vi "Remove Danger Move Options.vi"(5 "Danger Directions":T1[](array[typedef]), 7 "Danger View":i32[](array[numeric]), 10 "Danger Threshold":i32, 11 "Direction List":T1[](array[typedef])) -> (2 "Danger":bool, 3 "Safe Directions Out":T1[](array[typedef]))   [LabVIEW 2017, in "AntFarm_MB.lvclass"]
uses:
  AntFarm_MB.lvclass
  Type Defs/Direction Enum.ctl
  Type Defs/SB Type Defs.lvlib
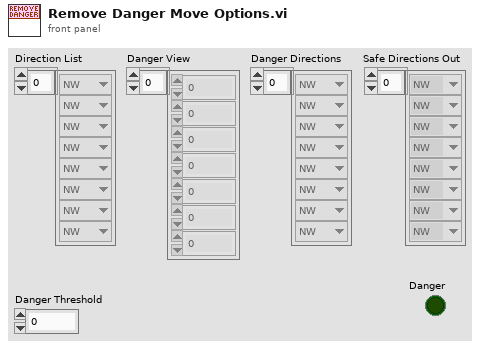
[diagram p1: front panel]
types:
  T1 = typedef "SB Type Defs.lvlib/Direction Enum.ctl" = enum16{"NW", "N", "NE", "E", "SE", "S", "SW", "W"}
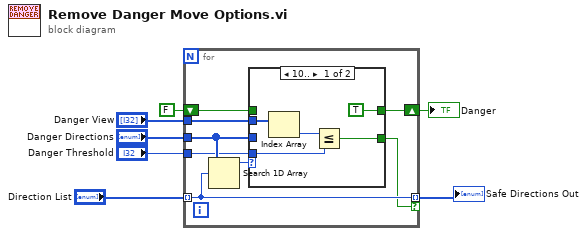
[diagram p0: block diagram]
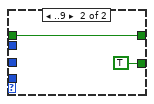
[diagram p2: hidden frame]
diagram:
  n1 = for {
    tunnel: "Direction List" -> [w13] mode=indexing
    tunnel: "Danger View" -> [w14]
    tunnel: "Danger Directions" -> [w12]
    tunnel: "Danger Threshold" -> [w11]
    tunnel: [w13] -> w7 mode=indexing if=w10
    shift-right: [w9] -> w1
    shift-left: FALSE -> [w8]
    n2 = Search 1D Array(1D array=w12, element=w13) -> (index of element=w15:i32)  [unwired: 1 in]
    n3 = case shown="10.." w15 {
      tunnel: w14 -> [w20 _]
      tunnel: w12 -> [_ _]
      tunnel: w11 -> [w18 _]
      tunnel: [w17 TRUE] -> w10
      tunnel: [TRUE w22] -> w9
      tunnel: w8 -> [_ w22]
      frame 10.. {
        n4 = Index Array(array=w20) -> (element=w19:i32)  [unwired: 1 in]
        n5 = Less Or Equal?(x=w19, y=w18) -> (x <= y?=w17:bool)
      }
      frame ..9 {
      }
    }
  }
  "Safe Directions Out" <- w7
  "Danger" <- w1
